vi "Python String to LabVIEW Data (U32 Array).vi"(8 "error in (no error)":errorcluster, 9 "type":u32[](array[numeric]), 10 "Python String":string) -> (0 "error out":errorcluster, 2 "LabVIEW Data":u32[](array[numeric]))   [LabVIEW 2020, in "jki_python_data_tools.lvlib"]
doc: "Reads a value associated with key in a specified section of the configuration data identified by refnum. If \"key\" input is not specified, the name of the variant object is used as the key. the \"found?\" output will be TRUE for compount objects (clusters) only if all elements (recursively) are found.\n\nFor example a Boolean named \"Enable\" with a value of TRUE would correspond to the key-value pair:\n\nEnable=TRUE"
uses:
  jki_python_data_tools.lvlib
  <userlib>/_OpenG.lib/string/string.llb/openg_string.lvlib
panel:
  # "Copyright © 2003-2009 JKI. All rights reserved.\n\nAuthor:\nPhilippe Guerit [philippe.guerit@jameskring.com]\nJim Kring [jim.kring@jameskring.com]\n\nThis library is provided \"AS IS\" ,WITHOUT WARRANTIES OR \nCONDITIONS OF ANY KIND, either express or implied.\n\nJames Kring, Inc. -- http://www.jameskring.com"
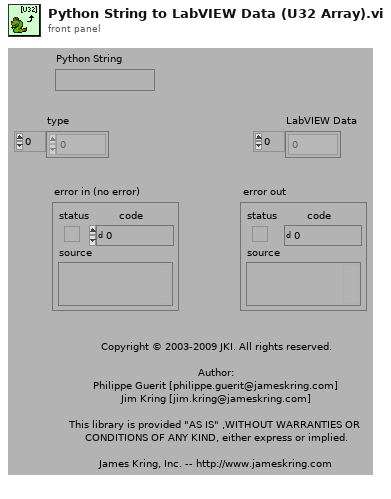
[diagram p1: front panel]
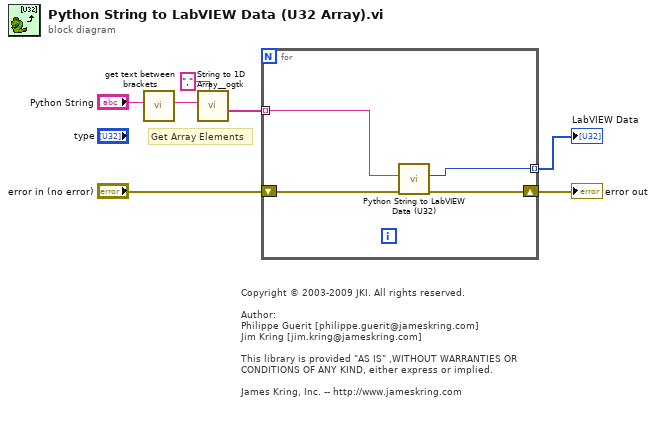
[diagram p0: block diagram]
diagram:
  # "Get Array Elements"
  # "Copyright © 2003-2009 JKI. All rights reserved.\n\nAuthor:\nPhilippe Guerit [philippe.guerit@jameskring.com]\nJim Kring [jim.kring@jameskring.com]\n\nThis library is provided \"AS IS\" ,WITHOUT WARRANTIES OR \nCONDITIONS OF ANY KIND, either express or implied.\n\nJames Kring, Inc. -- http://www.jameskring.com"
  n1 = call "get text between brackets.vi"("Python String"="Python String") -> ("Text Between Brakets"=w1:string)  [unwired: 10 in]
  n2 = call <userlib>:"String to 1D Array__ogtk.vi"("delimiter (Tab)"=",", "string"=w1) -> ("Array of Strings"=w6:string[])  [unwired: 9 in]
  n3 = for {
    tunnel: [w8] -> w3 mode=indexing
    tunnel: w6 -> [w11] mode=indexing
    shift-right: [w9] -> w4
    shift-left: "error in (no error)" -> [w10]
    n4 = call "Python String to LabVIEW Data (U32).vi"("error in (no error)"=w10, "Python String"=w11) -> ("error out"=w9:errorcluster, "LabVIEW Data"=w8:u32)  [unwired: 8 in]
  }
  "error out" <- w4
  "LabVIEW Data" <- w3
